vi "sliderFwBw.vi"(1 "mode":u16(ring) items=["fw", "bw"]) -> ()   [LabVIEW 2017]
uses:
  globalDevices.vi
  <vilib>/Instr/_visa.llb/VISA Flush IO Buffer Mask.ctl
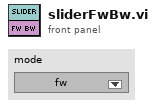
[diagram p1: front panel]
types:
  T1 = typedef "VISA Flush IO Buffer Mask.ctl" = u16
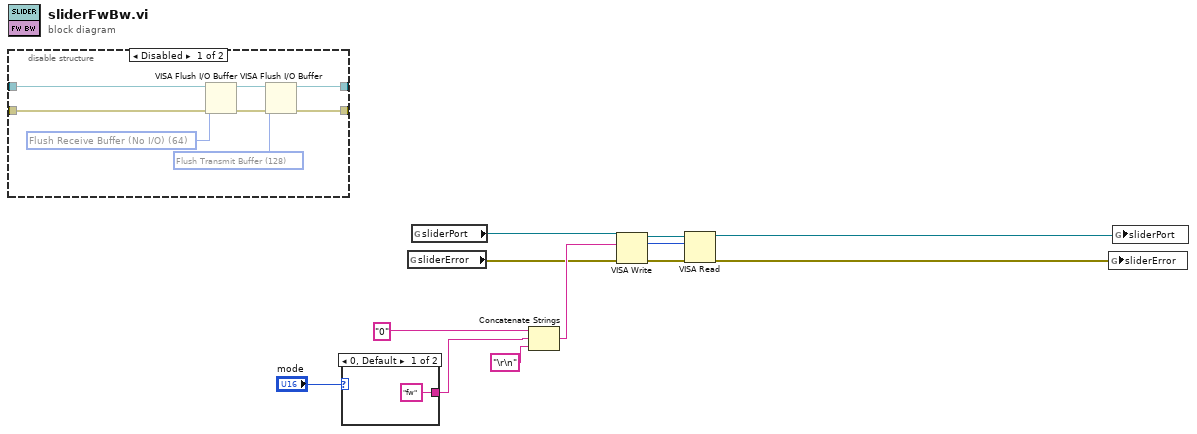
[diagram p0: block diagram]
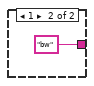
[diagram p3: hidden frame]
diagram:
  n1 = disable-structure shown="Disabled" {
    disable-tunnel: _ -> [w20 _]
    disable-tunnel: _ -> [w19 _]
    disable-tunnel: [w15 _] -> _
    disable-tunnel: [w14 _] -> _
    frame Disabled {
      w13 = T1 128 items=["Flush Receive Buffer"=16, "Write Transmit Buffer to Device"=32, "Flush Receive Buffer (No I/O)"=64, "Flush Transmit Buffer"=128] ("Mask")
      w18 = T1 64 items=["Flush Receive Buffer"=16, "Write Transmit Buffer to Device"=32, "Flush Receive Buffer (No I/O)"=64, "Flush Transmit Buffer"=128] ("Mask")
      n2 = VISA Flush I/O Buffer(VISA resource name=w20, mask (16)=w18, error in (no error)=w19) -> (VISA resource name out=w16:refnum<visa-resource-name>, error out=w17:errorcluster)
      n3 = VISA Flush I/O Buffer(VISA resource name=w16, mask (16)=w13, error in (no error)=w17) -> (VISA resource name out=w15:refnum<visa-resource-name>, error out=w14:errorcluster)
    }
    frame Enabled {
    }
  }
  n4 = case shown="0, Default" "mode" {
    tunnel: ["fw" "bw"] -> w4
    frame 0, Default {
    }
    frame 1 {
    }
  }
  n5 = global read "globalDevices.vi" "sliderError"() -> (w2:errorcluster)
  n6 = global read "globalDevices.vi" "sliderPort"() -> (w3:refnum<visa-resource-name>)
  n7 = Concatenate Strings("0", w4, "\r\n" ("string")) -> (w11:string)
  n8 = VISA Write(VISA resource name=w3, write buffer=w11, error in (no error)=w2) -> (VISA resource name out=w10:refnum<visa-resource-name>, return count=w9:u32, error out=w8:errorcluster)
  n9 = VISA Read(VISA resource name=w10, byte count=w9, error in (no error)=w8) -> (VISA resource name out=w7:refnum<visa-resource-name>, error out=w6:errorcluster)  [unwired: 2 out]
  n10 = global write "globalDevices.vi" "sliderError"(w6) -> ()
  n11 = global write "globalDevices.vi" "sliderPort"(w7) -> ()
